vi "Create Sysdef Tree from DB Channel Clusters_RTs.vi"(6 "broadcast":bool, 7 "Autocreate Rx timestamp chans?":bool, 8 "error in":errorcluster, 10 "RTs":T1[](array[typedef]), 11 "Device Ptr":u64) -> (0 "error out":errorcluster)   [LabVIEW 2020, in "Ballard 1553 System Explorer.lvlib"]
uses:
  Ballard 1553 System Explorer.lvlib
  Parse XML Ballard/Ballard_RT.ctl
  Parse XML Ballard/Ballard_RT subAddress.ctl
  Parse XML Ballard/Ballard_RT direction.ctl
  Parse XML Ballard/Ballard_RT rtMode.ctl
  Parse XML Ballard/Ballard_RT modeCode.ctl
  <vilib>/NI VeriStand/Custom Device API/Custom Device Channel.ctl
  <vilib>/NI VeriStand/Custom Device API/Custom Device Channel Type.ctl
  Shared/Controls and Global/Global.vi
  <vilib>/NI VeriStand/Custom Device API/Set Item Property (I32).vi
  <vilib>/NI VeriStand/Custom Device API/Set Item Property (U16).vi
  <vilib>/NI VeriStand/Custom Device API/Custom Device API.lvlib
  Shared/Ballard 1553 Shared.lvlib
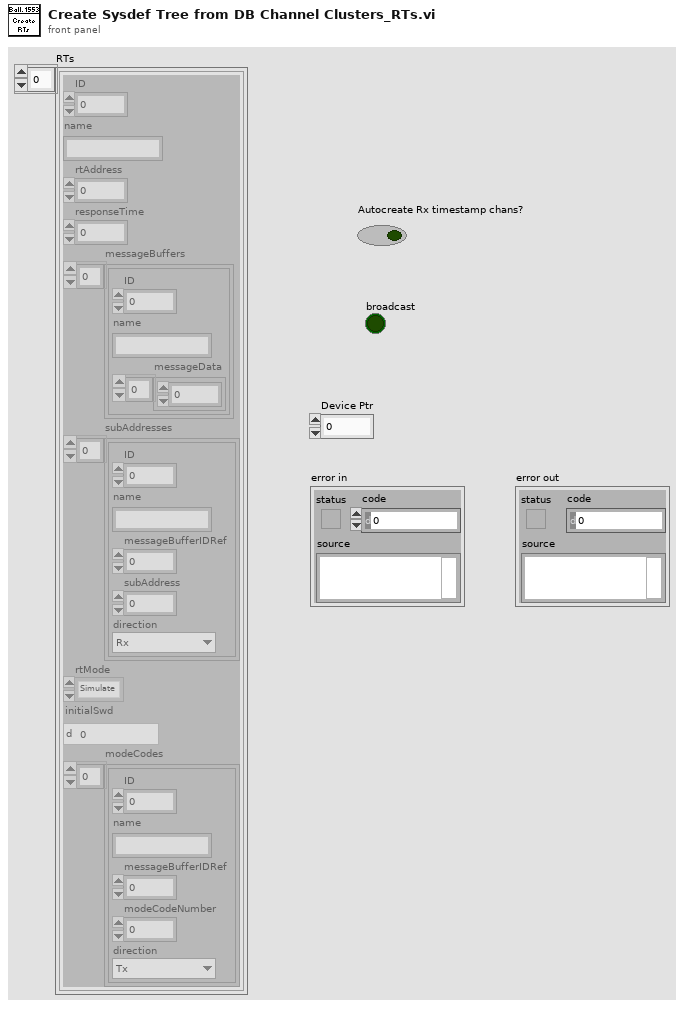
[diagram p1: front panel]
types:
  T1 = typedef "Ballard 1553 System Explorer.lvlib/Ballard_RT.ctl" = cluster{"ID":i32, "name":string, "rtAddress":i8, "responseTime":i32, "messageBuffers":cluster{"ID":i32, "name":string, "messageData":u16[]}[], "subAddresses":T2[], "rtMode":T4, "initialSwd":u16, "modeCodes":T5[]}
  T2 = typedef "Ballard 1553 System Explorer.lvlib/Ballard_RT subAddress.ctl" = cluster{"ID":i32, "name":string, "messageBufferIDRef":i32, "subAddress":i8, "direction":T3}
  T3 = typedef "Ballard 1553 System Explorer.lvlib/Ballard_RT direction.ctl" = enum16{"Tx", "Rx"}
  T4 = typedef "Ballard 1553 System Explorer.lvlib/Ballard_RT rtMode.ctl" = enum16{"Simulate", "Monitor", "Disable"}
  T5 = typedef "Ballard 1553 System Explorer.lvlib/Ballard_RT modeCode.ctl" = cluster{"ID":i32, "name":string, "messageBufferIDRef":i32, "modeCodeNumber":i8, "direction":T3}
  T6 = typedef "Custom Device API.lvlib/Custom Device Channel Type.ctl" = enum16{"Input", "Output"}
  T7 = typedef "Custom Device API.lvlib/Custom Device Channel.ctl" = cluster{"Type":T6, "Units":string, "Default Value":dbl, "Faultable":bool, "Scalable":bool}
  T8 = enum16{"DW", "STC", "SPC", "SW", "TI MC", "AC", "TI WC"}
  T9 = cluster{"ID":i32, "name":string, "messageData":u16[]}[]
  T10 = typedef "Custom Device API.lvlib/Custom Device Item Ref.ctl" = u64
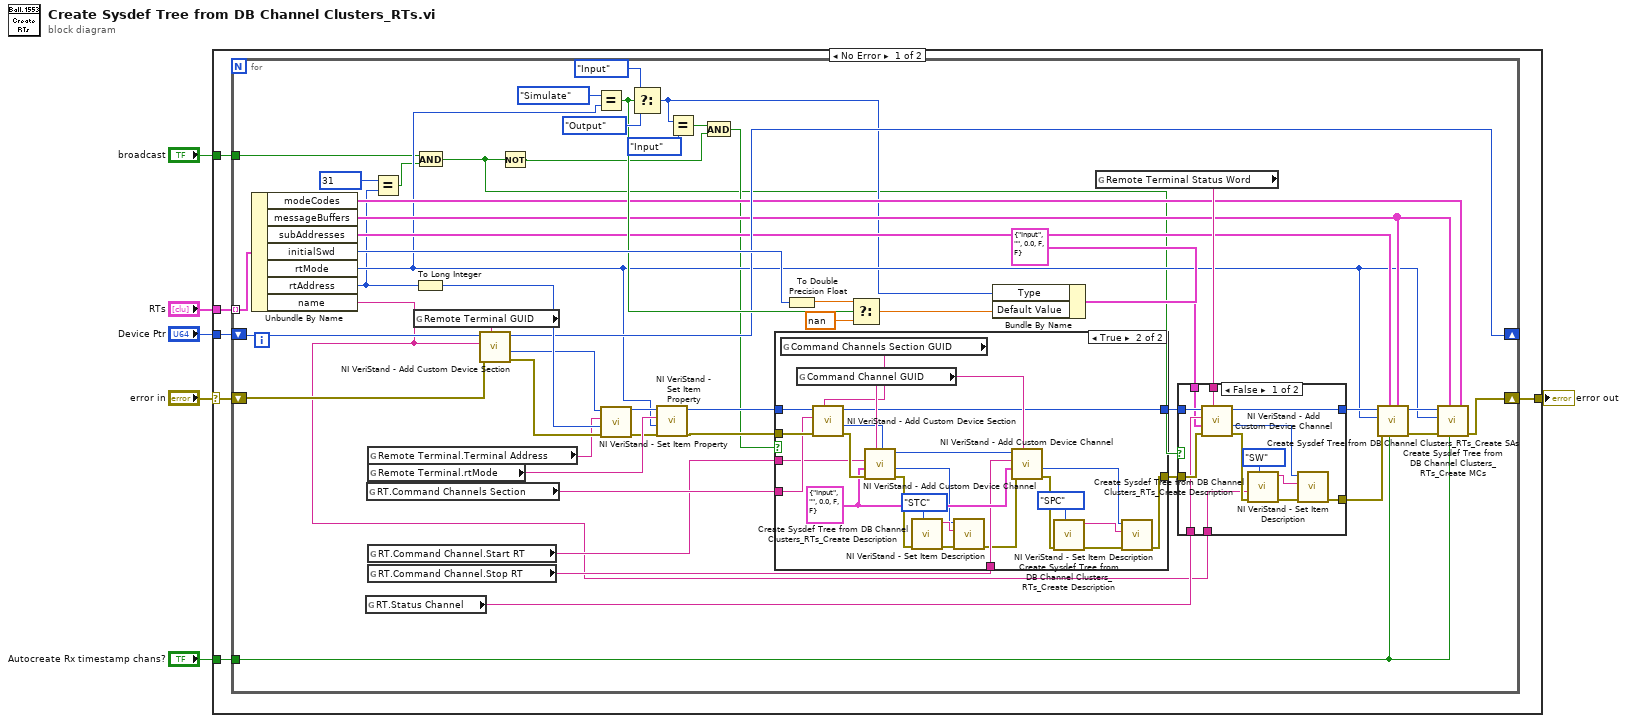
[diagram p0: block diagram]
diagram:
  n1 = case shown="No Error" "error in" {
    selector: "error in" -> [w11 w105]
    tunnel: [w10 w105] -> w5
    tunnel: "Device Ptr" -> [w12 _]
    tunnel: "RTs" -> [w8 _]
    tunnel: "Autocreate Rx timestamp chans?" -> [w9 _]
    tunnel: "broadcast" -> [w7 _]
    frame No Error {
      n2 = for {
        tunnel: w8 -> [w63] mode=indexing
        shift-right: [w30] -> w10
        shift-left: w11 -> [w36]
        tunnel: w9 -> [w25]
        shift-right: [w37] -> _
        shift-left: w12 -> [w35]
        tunnel: w7 -> [w20]
        n3 = Unbundle By Name(w63) -> ("modeCodes"=w28:T5[], "messageBuffers"=w29:T9, "subAddresses"=w31:T2[], "initialSwd"=w46:u16, "rtMode"=w27:T4, "rtAddress"=w22:i8, "name"=w23:string)
        n4 = global read "Global.vi" "RT.Status Channel"() -> (w49:string)
        n5 = global read "Global.vi" "RT.Command Channels Section"() -> (w54:string)
        n6 = global read "Global.vi" "Remote Terminal.Terminal Address"() -> (w59:string)
        n7 = global read "Global.vi" "Remote Terminal.rtMode"() -> (w57:string)
        n8 = global read "Global.vi" "RT.Command Channel.Start RT"() -> (w53:string)
        n9 = global read "Global.vi" "RT.Command Channel.Stop RT"() -> (w52:string)
        n10 = Equal?(x=i8 31, y=w22) -> (x = y?=w19:bool)
        n11 = global read "Global.vi" "Remote Terminal GUID"() -> (w62:string)
        n12 = To Long Integer(number=w22) -> (32bit integer=w60:i32)
        n13 = And(x=w20, y=w19) -> (x .and. y?=w13:bool)
        n14 = call <vilib>:"NI VeriStand - Add Custom Device Section.vi"("GUID (Default Section)"=w62, "error in (no error)"=w36, "Section Name"=w23, "Parent Ref in"=w35) -> ("error out"=w61:errorcluster, "Section Ptr"=w26:T10, "Parent Ref out"=w37:T10)  [unwired: 4 in, 1 out]
        n15 = Not(x=w13) -> (.not. x?=w14:bool)
        n16 = Equal?(x=Ballard_RT_rtMode."Simulate", y=w27) -> (x = y?=w39:bool)
        n17 = call-poly <vilib>:"NI VeriStand - Set Item Property.vi"("error in (no error)"=w61, "Value"=w60, "Property Name"=w59, "Item Ref in"=w26) -> ("error out"=w55:errorcluster, "Item Ref out"=w58:T10)  [unwired: 5 in, 1 out]
        n18 = Select(t=Custom_Device_Channel_Type."Input" ("Type"), s=w39, f=Custom_Device_Channel_Type."Output") -> (s? t:f=w18:T6)
        n19 = call-poly <vilib>:"NI VeriStand - Set Item Property.vi"("Value"=w27, "Property Name"=w57, "Item Ref in"=w58) -> ("Item Ref out"=w56:T10)  [unwired: 6 in, 2 out]
        n20 = Equal?(x=w18, y=Custom_Device_Channel_Type."Input") -> (x = y?=w16:bool)
        n21 = And(x=w16, y=w14) -> (x .and. y?=w15:bool)
        n22 = case shown="True" w15 {
          tunnel: w56 -> [w80 w99]
          tunnel: w55 -> [w79 w98]
          tunnel: w54 -> [_ w97]
          tunnel: w53 -> [_ w96]
          tunnel: w52 -> [_ w95]
          tunnel: [w80 w94] -> w51
          tunnel: [w79 w86] -> w50
          frame False {
            # "It's either a Monitor RT or broadcast RT."
          }
          frame True {
            w100 = T7 {"Type"=enum."Input", "Units"="", "Default Value"=0.0, "Faultable"=FALSE, "Scalable"=FALSE} ("Channel")
            n23 = global read "Global.vi" "Command Channels Section GUID"() -> (w93:string)
            n24 = global read "Global.vi" "Command Channel GUID"() -> (w104:string)
            n25 = call <vilib>:"NI VeriStand - Add Custom Device Section.vi"("GUID (Default Section)"=w93, "error in (no error)"=w98, "Section Name"=w97, "Parent Ref in"=w99) -> ("error out"=w102:errorcluster, "Section Ptr"=w101:T10, "Parent Ref out"=w94:T10)  [unwired: 4 in, 1 out]
            n26 = call <vilib>:"NI VeriStand - Add Custom Device Channel.vi"("GUID (Default Channel)"=w104, "error in (no error)"=w102, "Channel"=w100, "Channel Name"=w96, "Parent Ref in"=w101) -> ("error out"=w92:errorcluster, "Channel Ref"=w84:T10, "Parent Ref out"=w103:T10)  [unwired: 3 in, 1 out]
            n27 = call "Create Sysdef Tree from DB Channel Clusters_RTs_Create Description.vi"("Type"=T8."STC", "error in (no error)"=w92) -> ("error out"=w91:errorcluster, "Description (Out)"=w90:string)  [unwired: 8 in]
            n28 = call <vilib>:"NI VeriStand - Set Item Description.vi"("error in (no error)"=w91, "Description"=w90, "Item Ref in"=w84) -> ("error out"=w85:errorcluster)  [unwired: 6 in, 2 out]
            n29 = call <vilib>:"NI VeriStand - Add Custom Device Channel.vi"("GUID (Default Channel)"=w104, "error in (no error)"=w85, "Channel"=w100, "Channel Name"=w95, "Parent Ref in"=w103) -> ("error out"=w87:errorcluster, "Channel Ref"=w83:T10)  [unwired: 3 in, 2 out]
            n30 = call "Create Sysdef Tree from DB Channel Clusters_RTs_Create Description.vi"("Type"=T8."SPC", "error in (no error)"=w87) -> ("error out"=w88:errorcluster, "Description (Out)"=w89:string)  [unwired: 8 in]
            n31 = call <vilib>:"NI VeriStand - Set Item Description.vi"("error in (no error)"=w88, "Description"=w89, "Item Ref in"=w83) -> ("error out"=w86:errorcluster)  [unwired: 6 in, 2 out]
          }
        }
        n32 = To Double Precision Float(number=w46) -> (double precision float=w40:dbl)
        n33 = Select(t=w40, s=w39, f=nan) -> (s? t:f=w41:dbl)
        n34 = Bundle By Name(cluster=T7 {"Type"=enum."Input", "Units"="", "Default Value"=0.0, "Faultable"=FALSE, "Scalable"=FALSE} ("Channel"), "Type"=w18, "Default Value"=w41) -> (w47:T7)
        n35 = global read "Global.vi" "Remote Terminal Status Word"() -> (w45:string)
        n36 = case shown="False" w13 {
          tunnel: w51 -> [w76 w78]
          tunnel: w50 -> [w75 w77]
          tunnel: w49 -> [w74 _]
          tunnel: w47 -> [w73 _]
          tunnel: w45 -> [w72 _]
          tunnel: [w71 w78] -> w32
          tunnel: [w67 w77] -> w24
          tunnel: w23 -> [w65 _]
          frame False {
            n37 = call <vilib>:"NI VeriStand - Add Custom Device Channel.vi"("GUID (Default Channel)"=w72, "error in (no error)"=w75, "Channel"=w73, "Channel Name"=w74, "Parent Ref in"=w76) -> ("error out"=w69:errorcluster, "Channel Ref"=w66:T10, "Parent Ref out"=w71:T10)  [unwired: 3 in, 1 out]
            n38 = call "Create Sysdef Tree from DB Channel Clusters_RTs_Create Description.vi"("Type"=T8."SW", "error in (no error)"=w69, "Name"=w65) -> ("error out"=w70:errorcluster, "Description (Out)"=w68:string)  [unwired: 7 in]
            n39 = call <vilib>:"NI VeriStand - Set Item Description.vi"("error in (no error)"=w70, "Description"=w68, "Item Ref in"=w66) -> ("error out"=w67:errorcluster)  [unwired: 6 in, 2 out]
          }
          frame True {
            # "It's the broadcast RT\nThere is no Status for it."
          }
        }
        n40 = call "Create Sysdef Tree from DB Channel Clusters_RTs_Create SAs.vi"("messageBuffers"=w29, "Autocreate Rx timestamp chans?"=w25, "subAddresses"=w31, "error in (no error)"=w24, "rtMode"=w27, "Section Ptr in"=w32) -> ("error out"=w34:errorcluster, "Section Ptr out"=w33:T10)  [unwired: 4 in]
        n41 = call "Create Sysdef Tree from DB Channel Clusters_RTs_Create MCs.vi"("modeCodes"=w28, "Autocreate Rx timestamp chans?"=w25, "messageBuffers"=w29, "error in (no error)"=w34, "rtMode"=w27, "Section Ptr in"=w33) -> ("error out"=w30:errorcluster)  [unwired: 5 in]
      }
    }
    frame Error {
    }
  }
  "error out" <- w5
